vi "Configuration Parse.vi"(8 "error in":errorcluster, 11 "UI Control":T8={"measurement configuration"={"Automation Test"=FALSE, "Power sequencing file path"="", "RFSG name"="", "RFSG port"="", "RFSG attenuation mode"=enum."<None>", "RFSG external attenuation (dB)"=0.0, "RFSG s-parameters orientation"=enum."Port1 Towards DUT", "RFSG s2p file path"="", "RFmx name"="", "RFmx port"="", "RFmx attenuation mode"=enum."<None>", "RFmx external attenuation (dB)"=0.0, "RFmx s-parameters orientation"=enum."Port1 Towards DUT", "RFmx s2p file path"="", "RFmx Reference Level (dBm)"=0.0, "RFSG Generation IQ Rate (S/s)"=0.0, "Target Pout Per Tone (dBm)"=0.0, "Start Pin Per Tone (dBm)"=0.0, "Start Center Frequency (Hz)"=0.0, "Start Tone Spacing (Hz)"=0.0, "IM_Sweep Mode"=enum."Power", "Sweep Delay (ms)"=0, "Power Sweep End"=0.0, "Power Sweep Step"=0.0, "Frequency Sweep End"=-4.0, "Frequency Sweep Step"=1.0, "Tone Spacing Sweep End"=-4.0, "Tone Spacing Sweep Step"=1.0}, "measurement results"={"Status"="", "Typical OIP3 (dBm)"=0.0, "TS_Fundamental (dBm)"=[], "TS_IMD (dBm)"=[], "TS_TOI (dBm)"=[], "TS_DUT Gain (dBm)"=[], "TS_Fundamental Slope (dBm)"=[], "TS_Intermodulation Slope (dBm)"=[], "Final Target Pout (dBm)"=0.0}} {"measurement configuration"."Tone Spacing Sweep Step" format="%#.pHz"; "measurement configuration"."Tone Spacing Sweep End" format="%#.pHz"; "measurement configuration"."Frequency Sweep Step" format="%#.pHz"; "measurement configuration"."Frequency Sweep End" format="%#.pHz"; "measurement configuration"."Power Sweep End" format="%#.6f"; "measurement configuration"."Sweep Delay (ms)" format="%#.6f"; "measurement configuration"."Start Tone Spacing (Hz)" format="%#.6p"; "measurement configuration"."Start Center Frequency (Hz)" format="%#.6p"; "measurement configuration"."Start Pin Per Tone (dBm)" format="%#.6p"; "measurement configuration"."Target Pout Per Tone (dBm)" format="%#.6f"; "measurement configuration"."RFSG Generation IQ Rate (S/s)" format="%#.6f"; "measurement configuration"."RFmx Reference Level (dBm)" format="%#_6p"; "measurement configuration"."RFmx external attenuation (dB)" format="%.2f"; "measurement configuration"."RFSG external attenuation (dB)" format="%.2f"}) -> (0 "error out":errorcluster, 1 "RFmx Settings":T1={"Reference Level (dBm)"=20.0, "Attenuation"={"RFmx Name"="", "RFmx Port"="", "Attenuation"={"Mode"=enum."Constant Attenuation", "Constant Attenuation"={"RFmx External Attenuation (dB)"=1.2}, "s2p File"={"RFmx S-Parameters Orientation"=24000, "RFmx Attenuation s2p Path Name"="", "RFmx Attenuation s2p File"=path ""}}}} {"Attenuation"."Attenuation"."s2p File"."RFmx S-Parameters Orientation" items=["Port1 Towards DUT"=24000, "Port2 Towards DUT"=24001]; "Attenuation"."Attenuation"."Constant Attenuation"."RFmx External Attenuation (dB)" format="%.2f"; "Reference Level (dBm)" format="%.2f"}, 2 "RFSG Settings":T3={"IQ Rate (S/sec)"=10000000.0, "Number of Samples"=3000, "Attenuation"={"RFSG Name"="5842_0", "RFSG Port"="", "Attenuation"={"Mode"=enum."Constant Attenuation", "Contant Attenuation"={"RFSG External Attenuation (dB)"=2.0}, "s2p File"={"RFSG S-parameters Orientation"=24000, "RFSG Attenuation s2p Path Name"="", "RFSG s2p File Path"=path ""}}}} {"Attenuation"."Attenuation"."s2p File"."RFSG S-parameters Orientation" items=["Port1 Towards DUT"=24000, "Port2 Towards DUT"=24001]; "Attenuation"."Attenuation"."Contant Attenuation"."RFSG External Attenuation (dB)" format="%.2f"; "IQ Rate (S/sec)" format="%#.3p"}, 3 "Test Configuration":T5={"Target Pout Per Tone (dBm)"=0.0, "Start Value"={"Power Level per Tone (dBm)"=-20.0, "Center Frequency (Hz)"=10000000000.0, "Tone Spacing (Hz)"=1000000.0}, "Sweep Settings"={"Mode"=enum."Power", "Sweep Delay (ms)"=0, "Power Sweep End"=-20.0, "Power Sweep Step"=-20.0, "Frequency Sweep End"=-4.0, "Frequency Sweep Step"=1.0, "Tone Spacing Sweep End"=-4.0, "Tone Spacing Sweep Step"=1.0}} {"Sweep Settings"."Tone Spacing Sweep Step" format="%#.pHz"; "Sweep Settings"."Tone Spacing Sweep End" format="%#.pHz"; "Sweep Settings"."Frequency Sweep Step" format="%#.pHz"; "Sweep Settings"."Frequency Sweep End" format="%#.pHz"; "Start Value"."Tone Spacing (Hz)" format="%#_6p"; "Start Value"."Center Frequency (Hz)" format="%#.3p"})   [LabVIEW 2023, in "FPT Intermodulation.lvclass"]
uses:
  FPT Intermodulation.lvclass
  FPT Intermodulation.lvclass/FPT Intermodulation.ctl
  Measurement/Controls/RFSG Config - TOI.ctl
  Measurement/Controls/RFmx Config - TOI.ctl
  Measurement/Controls/Test Config - TOI.ctl
  FPT Shared VIs/De-embedding/RFsg Config.ctl
  FPT Shared VIs/De-embedding/RFmx Config.ctl
  Measurement Configuration.ctl
  Measurement Results.ctl
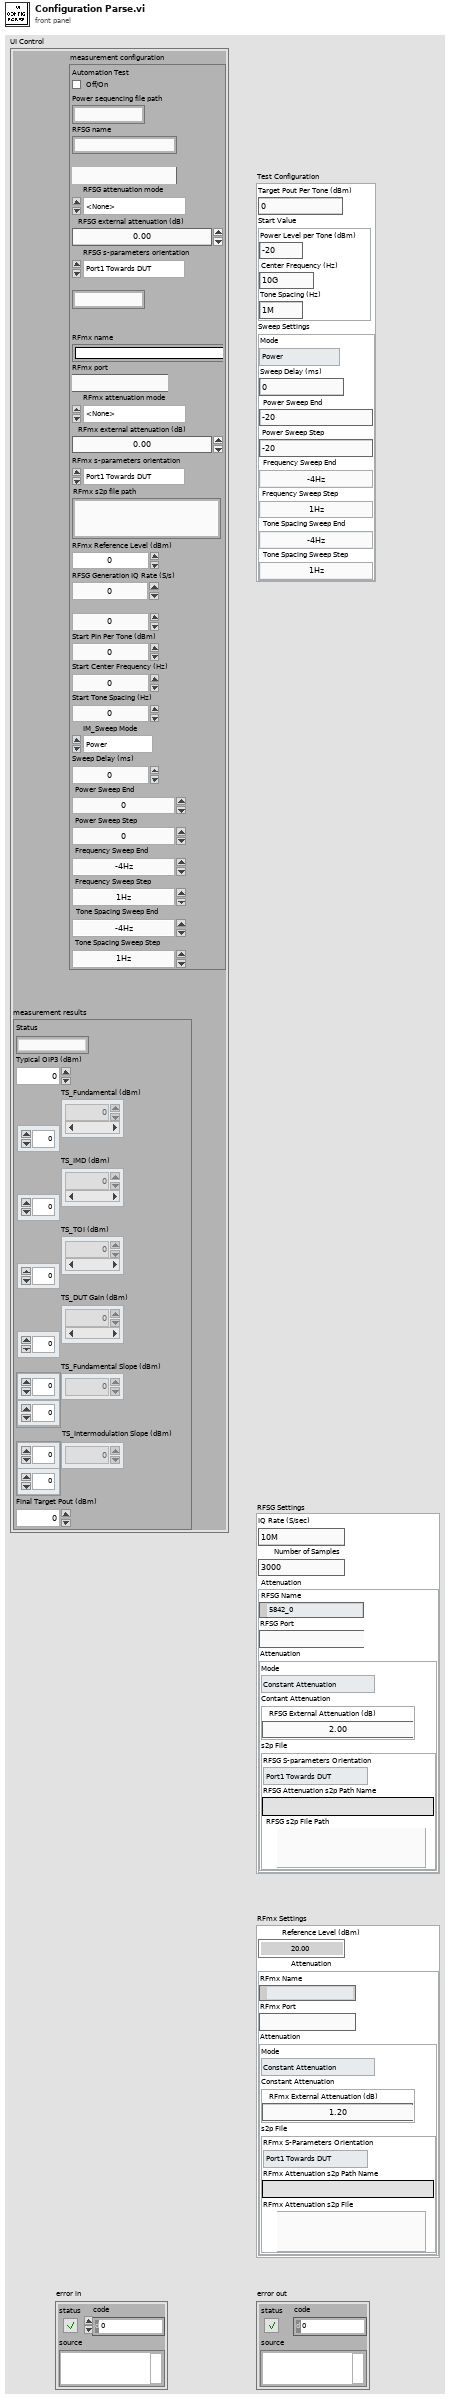
[diagram p1: front panel]
types:
  T1 = typedef "RFmx Config - TOI.ctl" = cluster{"Reference Level (dBm)":dbl, "Attenuation":T2}
  T2 = typedef "RFmx Config.ctl" = cluster{"RFmx Name":refnum<k15>, "RFmx Port":string, "Attenuation":cluster{"Mode":enum32{"<None>", "Constant Attenuation", "s2p File"}, "Constant Attenuation":cluster{"RFmx External Attenuation (dB)":dbl}, "s2p File":cluster{"RFmx S-Parameters Orientation":i32, "RFmx Attenuation s2p Path Name":string, "RFmx Attenuation s2p File":path}}}
  T3 = typedef "RFSG Config - TOI.ctl" = cluster{"IQ Rate (S/sec)":dbl, "Number of Samples":i32, "Attenuation":T4}
  T4 = typedef "RFsg Config.ctl" = cluster{"RFSG Name":refnum<k15>, "RFSG Port":string, "Attenuation":cluster{"Mode":enum32{"<None>", "Constant Attenuation", "s2p File"}, "Contant Attenuation":cluster{"RFSG External Attenuation (dB)":dbl}, "s2p File":cluster{"RFSG S-parameters Orientation":i32, "RFSG Attenuation s2p Path Name":string, "RFSG s2p File Path":path}}}
  T5 = typedef "Test Config - TOI.ctl" = cluster{"Target Pout Per Tone (dBm)":dbl, "Start Value":cluster{"Power Level per Tone (dBm)":dbl, "Center Frequency (Hz)":dbl, "Tone Spacing (Hz)":dbl}, "Sweep Settings":cluster{"Mode":enum16{"Power", "Frequency", "Tone Spacing"}, "Sweep Delay (ms)":u32, "Power Sweep End":dbl, "Power Sweep Step":dbl, "Frequency Sweep End":dbl, "Frequency Sweep Step":dbl, "Tone Spacing Sweep End":dbl, "Tone Spacing Sweep Step":dbl}}
  T6 = typedef "FPT Intermodulation.lvclass/Measurement Configuration.ctl" = cluster{"Automation Test":bool, "Power sequencing file path":string, "RFSG name":string, "RFSG port":string, "RFSG attenuation mode":enum32{"<None>", "Constant Attenuation", "s2p File"}, "RFSG external attenuation (dB)":dbl, "RFSG s-parameters orientation":enum32{"Port1 Towards DUT", "Port2 Towards DUT"}, "RFSG s2p file path":string, "RFmx name":string, "RFmx port":string, "RFmx attenuation mode":enum32{"<None>", "Constant Attenuation", "s2p File"}, "RFmx external attenuation (dB)":dbl, "RFmx s-parameters orientation":enum32{"Port1 Towards DUT", "Port2 Towards DUT"}, "RFmx s2p file path":string, "RFmx Reference Level (dBm)":dbl, "RFSG Generation IQ Rate (S/s)":dbl, "Target Pout Per Tone (dBm)":dbl, "Start Pin Per Tone (dBm)":dbl, "Start Center Frequency (Hz)":dbl, "Start Tone Spacing (Hz)":dbl, "IM_Sweep Mode":enum32{"Power", "Frequency", "Tone Spacing"}, "Sweep Delay (ms)":u32, "Power Sweep End":dbl, "Power Sweep Step":dbl, "Frequency Sweep End":dbl, "Frequency Sweep Step":dbl, "Tone Spacing Sweep End":dbl, "Tone Spacing Sweep Step":dbl}
  T7 = typedef "FPT Intermodulation.lvclass/Measurement Results.ctl" = cluster{"Status":string, "Typical OIP3 (dBm)":dbl, "TS_Fundamental (dBm)":dbl[][], "TS_IMD (dBm)":dbl[][], "TS_TOI (dBm)":dbl[][], "TS_DUT Gain (dBm)":dbl[][], "TS_Fundamental Slope (dBm)":dbl[][], "TS_Intermodulation Slope (dBm)":dbl[][], "Final Target Pout (dBm)":dbl}
  T8 = cluster{"measurement configuration":T6, "measurement results":T7}
  T9 = enum32{"<None>", "Constant Attenuation", "s2p File"}
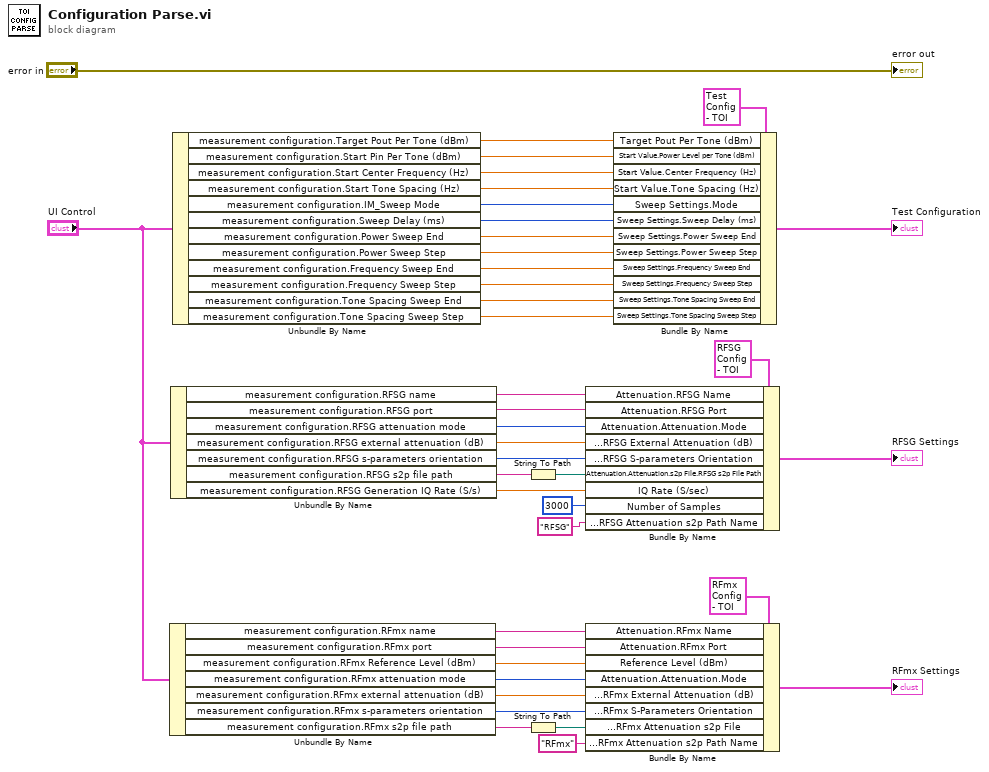
[diagram p0: block diagram]
diagram:
  n1 = Unbundle By Name("UI Control") -> ("measurement configuration.RFmx name"=w29:string, "measurement configuration.RFmx port"=w28:string, "measurement configuration.RFmx Reference Level (dBm)"=w27:dbl, "measurement configuration.RFmx attenuation mode"=w26:T9, "measurement configuration.RFmx external attenuation (dB)"=w25:dbl, "measurement configuration.RFmx s-parameters orientation"=w24:enum32{"Port1 Towards DUT", "Port2 Towards DUT"}, "measurement configuration.RFmx s2p file path"=w23:string)
  n2 = Unbundle By Name("UI Control") -> ("measurement configuration.RFSG name"=w38:string, "measurement configuration.RFSG port"=w9:string, "measurement configuration.RFSG attenuation mode"=w37:T9, "measurement configuration.RFSG external attenuation (dB)"=w36:dbl, "measurement configuration.RFSG s-parameters orientation"=w35:enum32{"Port1 Towards DUT", "Port2 Towards DUT"}, "measurement configuration.RFSG s2p file path"=w34:string, "measurement configuration.RFSG Generation IQ Rate (S/s)"=w20:dbl)
  n3 = Unbundle By Name("UI Control") -> ("measurement configuration.Target Pout Per Tone (dBm)"=w18:dbl, "measurement configuration.Start Pin Per Tone (dBm)"=w17:dbl, "measurement configuration.Start Center Frequency (Hz)"=w16:dbl, "measurement configuration.Start Tone Spacing (Hz)"=w15:dbl, "measurement configuration.IM_Sweep Mode"=w14:enum32{"Power", "Frequency", "Tone Spacing"}, "measurement configuration.Sweep Delay (ms)"=w12:u32, "measurement configuration.Power Sweep End"=w6:dbl, "measurement configuration.Power Sweep Step"=w5:dbl, "measurement configuration.Frequency Sweep End"=w4:dbl, "measurement configuration.Frequency Sweep Step"=w3:dbl, "measurement configuration.Tone Spacing Sweep End"=w2:dbl, "measurement configuration.Tone Spacing Sweep Step"=w1:dbl)
  n4 = String To Path(string=w34) -> (path=w33:path)
  n5 = String To Path(string=w23) -> (path=w22:path)
  n6 = Bundle By Name(cluster=T3 {"IQ Rate (S/sec)"=0.0, "Number of Samples"=0, "Attenuation"={"RFSG Name"="", "RFSG Port"="", "Attenuation"={"Mode"=enum."Constant Attenuation", "Contant Attenuation"={"RFSG External Attenuation (dB)"=0.0}, "s2p File"={"RFSG S-parameters Orientation"=24000, "RFSG Attenuation s2p Path Name"="", "RFSG s2p File Path"=path ""}}}} ("RFSG Settings"), "Attenuation.RFSG Name"=w38, "Attenuation.RFSG Port"=w9, "Attenuation.Attenuation.Mode"=w37, "Attenuation.Attenuation.Contant Attenuation.RFSG External Attenuation (dB)"=w36, "Attenuation.Attenuation.s2p File.RFSG S-parameters Orientation"=w35, "Attenuation.Attenuation.s2p File.RFSG s2p File Path"=w33, "IQ Rate (S/sec)"=w20, "Number of Samples"=3000, "Attenuation.Attenuation.s2p File.RFSG Attenuation s2p Path Name"="RFSG") -> (→"RFSG Settings":T3)
  n7 = Bundle By Name(cluster=T1 {"Reference Level (dBm)"=0.0, "Attenuation"={"RFmx Name"="", "RFmx Port"="", "Attenuation"={"Mode"=enum."Constant Attenuation", "Constant Attenuation"={"RFmx External Attenuation (dB)"=0.0}, "s2p File"={"RFmx S-Parameters Orientation"=24000, "RFmx Attenuation s2p Path Name"="", "RFmx Attenuation s2p File"=path ""}}}} ("RFmx Settings"), "Attenuation.RFmx Name"=w29, "Attenuation.RFmx Port"=w28, "Reference Level (dBm)"=w27, "Attenuation.Attenuation.Mode"=w26, "Attenuation.Attenuation.Constant Attenuation.RFmx External Attenuation (dB)"=w25, "Attenuation.Attenuation.s2p File.RFmx S-Parameters Orientation"=w24, "Attenuation.Attenuation.s2p File.RFmx Attenuation s2p File"=w22, "Attenuation.Attenuation.s2p File.RFmx Attenuation s2p Path Name"="RFmx") -> (→"RFmx Settings":T1)
  n8 = Bundle By Name(cluster=T5 {"Target Pout Per Tone (dBm)"=0.0, "Start Value"={"Power Level per Tone (dBm)"=-20.0, "Center Frequency (Hz)"=10000000000.0, "Tone Spacing (Hz)"=1000000.0}, "Sweep Settings"={"Mode"=enum."Power", "Sweep Delay (ms)"=0, "Power Sweep End"=1.0, "Power Sweep Step"=-4.0, "Frequency Sweep End"=-4.0, "Frequency Sweep Step"=1.0, "Tone Spacing Sweep End"=-4.0, "Tone Spacing Sweep Step"=1.0}} ("Test Configuration"), "Target Pout Per Tone (dBm)"=w18, "Start Value.Power Level per Tone (dBm)"=w17, "Start Value.Center Frequency (Hz)"=w16, "Start Value.Tone Spacing (Hz)"=w15, "Sweep Settings.Mode"=w14, "Sweep Settings.Sweep Delay (ms)"=w12, "Sweep Settings.Power Sweep End"=w6, "Sweep Settings.Power Sweep Step"=w5, "Sweep Settings.Frequency Sweep End"=w4, "Sweep Settings.Frequency Sweep Step"=w3, "Sweep Settings.Tone Spacing Sweep End"=w2, "Sweep Settings.Tone Spacing Sweep Step"=w1) -> (→"Test Configuration":T5)
  "error out" <- "error in"
